vi "Plural.vi"(10 "String":string) -> (2 "Plural":string)   [LabVIEW 2020, in "Conditum-Tools.lvlib"]
uses:
  Conditum-Tools.lvlib
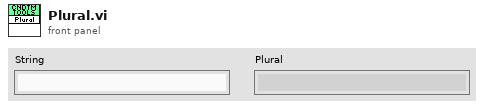
[diagram p1: front panel]
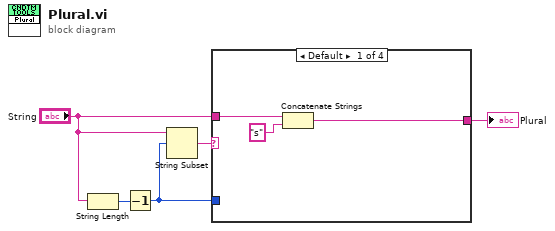
[diagram p0: block diagram]
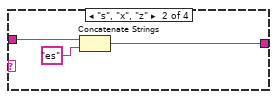
[diagram p2: hidden frame]
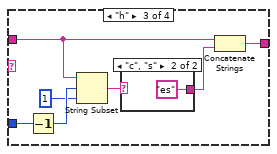
[diagram p3: hidden frame]
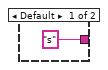
[diagram p4: hidden frame]
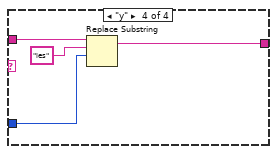
[diagram p5: hidden frame]
diagram:
  n1 = String Length(string="String") -> (length=w5:i32)
  n2 = Decrement(x=w5) -> (x-1=w1:i32)
  n3 = String Subset(string="String", offset (0)=w1) -> (substring=w3:string)  [unwired: 1 in]
  n4 = case shown="Default" w3 {
    tunnel: "String" -> [w8 w11 w14 w24]
    tunnel: [w6 w9 w13 w21] -> w2
    tunnel: w1 -> [_ _ w18 w23]
    frame Default {
      n5 = Concatenate Strings(w8, "s" ("string")) -> (w6:string)
    }
    frame "s", "x", "z" {
      n6 = Concatenate Strings(w11, "es" ("string")) -> (w9:string)
    }
    frame "h" {
      n7 = Decrement(x=w18) -> (x-1=w17:i32)
      n8 = String Subset(string=w14, offset (0)=w17, length (rest)=1 ("length (rest)")) -> (substring=w15:string)
      n9 = case shown="\"c\", \"s\"" w15 {
        tunnel: ["s" "es"] -> w12
        frame Default {
        }
        frame "c", "s" {
        }
      }
      n10 = Concatenate Strings(w14, w12) -> (w13:string)
    }
    frame "y" {
      n11 = Replace Substring(3:w23, 4:"ies" ("substring (\"\")"), 5:w24) -> (1:w21:string)  [unwired: 1 in, 1 out]
    }
  }
  "Plural" <- w2
